vi "Define Correlator Port.vi"(1 "VISA resource name":refnum<visa-resource-name>="COM1", 2 "Addr (0-15)":i8 min=0 max=15 step=1) -> ()   [LabVIEW 2012]
uses:
  Correlator port.vi
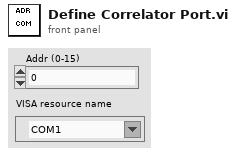
[diagram p1: front panel]
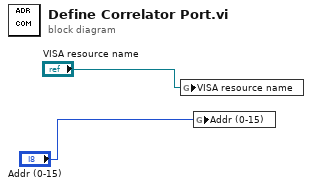
[diagram p0: block diagram]
diagram:
  n1 = global write "Correlator port.vi" "VISA resource name"("VISA resource name") -> ()
  n2 = global write "Correlator port.vi" "Addr (0-15)"("Addr (0-15)") -> ()
